vi "CalcDistance.vi"(9 "Distance In":u32 max=0 step=1, 10 "Accel In":u32, 11 "Speed In":i32) -> (1 "Distance Out":i32, 2 "Accel Out":u32, 3 "Speed Out":i32)   [LabVIEW 2015, in "Ion Motion Roboclaw.lvlib"]
uses:
  <instrlib>/Ion Motion Roboclaw/Ion Motion Roboclaw.lvlib
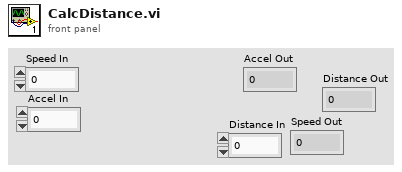
[diagram p1: front panel]
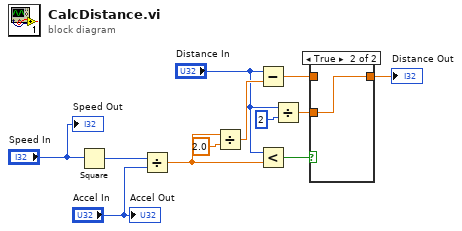
[diagram p0: block diagram]
diagram:
  n1 = Square(x="Speed In") -> (x^2=w12:i32)
  n2 = Divide(x=w12, y="Accel In") -> (x/y=w10:dbl)
  n3 = Divide(x=w10, y=2.0) -> (x/y=w9:dbl)
  n4 = Subtract(x="Distance In", y=w9) -> (x-y=w4:dbl)
  n5 = Less?(x="Distance In", y=w10) -> (x < y?=w6:bool)
  n6 = Divide(x="Distance In", y=u32 2) -> (x/y=w5:dbl)
  n7 = case shown="True" w6 {
    tunnel: [w13 w14] -> w3
    tunnel: w5 -> [_ w14]
    tunnel: w4 -> [w13 _]
    frame False {
    }
    frame True {
    }
  }
  "Distance Out" <- w3
  "Accel Out" <- "Accel In"
  "Speed Out" <- "Speed In"
